vi "Send2DGotoPos.vi"(8 "error in (no error)":errorcluster caption="entrée d'erreur (pas d'erreur)", 9 "GotoPos":dbl, 10 "InstrIndex":i32, 11 "Experiment en entrée":refnum<class "Experiment.lvclass"> caption="DNL_LabVIEW Object in") -> (0 "error out":errorcluster caption="sortie d'erreur", 3 "Experiment en sortie":refnum<class "Experiment.lvclass"> caption="DNL_LabVIEW Object out")   [LabVIEW 2019, in "Experiment.lvclass"]
uses:
  Experiment.lvclass
  DevicesClass/BaseDevice/ClassQueueMess.ctl
  Experiment.lvclass/Experiment.ctl
  DevicesClass/BaseDevice/BaseDevice.lvclass
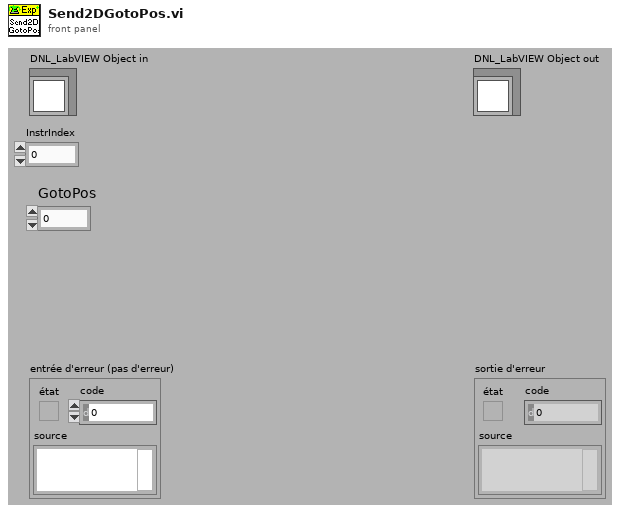
[diagram p1: front panel]
types:
  T1 = typedef "ClassQueueMess.ctl" = u16
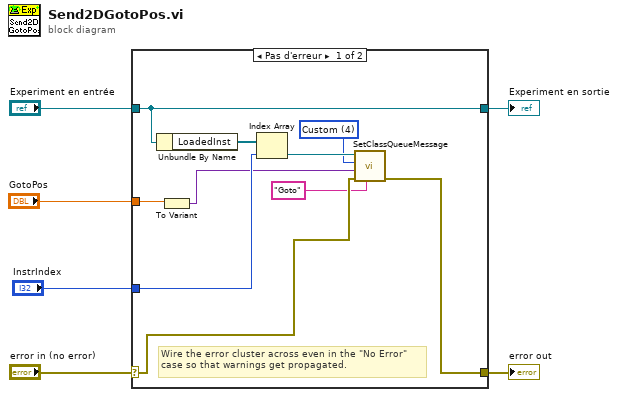
[diagram p0: block diagram]
diagram:
  n1 = case shown="Pas d'erreur" "error in (no error)" {
    selector: "error in (no error)" -> [w12 w18]
    tunnel: [w10 w18] -> w5
    tunnel: [w16 w17] -> w3
    tunnel: "Experiment en entrée" -> [w16 w17]
    tunnel: "InstrIndex" -> [w14 _]
    tunnel: "GotoPos" -> [w8 _]
    frame No Error {
      w11 = T1 4 items=["UpdateClassData", "UpdateMainClass", "UpdateDataBind", "ReInitDevice", "Custom", "ClosePan"] ("Menu déroulant")
      # "Wire the error cluster across even in the \"No Error\"\ncase so that warnings get propagated."
      n2 = Unbundle By Name(w16) -> ("LoadedInst"=w15:refnum<class "BaseDevice.lvclass">[])
      n3 = To Variant(anything=w8) -> (Variant=w7:variant)
      n4 = Index Array(array=w15, index=w14) -> (element=w13:refnum<class "BaseDevice.lvclass">)
      n5 = call-dynamic "SetClassQueueMessage.vi"("QMessage"="Goto", "ErrorIn(No Error)"=w12, "Data"=w7, "Menu déroulant"=w11, "BaseDevice.lvclass"=w13) -> ("sortie d'erreur"=w10:errorcluster)  [unwired: 5 in, 1 out]
    }
    frame Error {
    }
  }
  "error out" <- w5
  "Experiment en sortie" <- w3
